vi "Access Privilege_DeleteUser.vi"(8 "error in":errorcluster, 9 "File Path":path, 10 "Username":string, 11 "User ID Refnum":refnum<vi>) -> (0 "error out":errorcluster, 3 "Message Output":string)   [LabVIEW 2023, in "GUI.lvlib"]
doc: "This VI shall delete the selected user on confirmation"
uses:
  GUI.lvlib
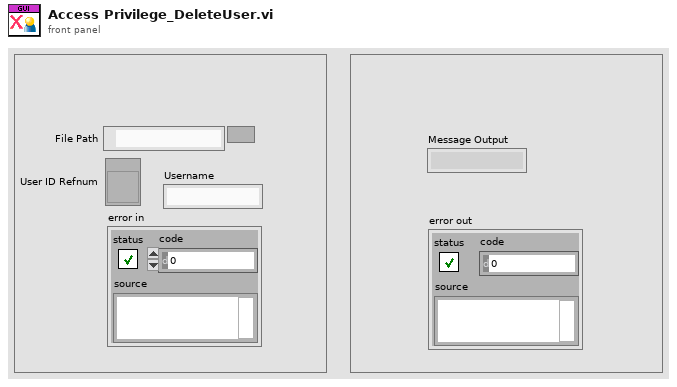
[diagram p1: front panel]
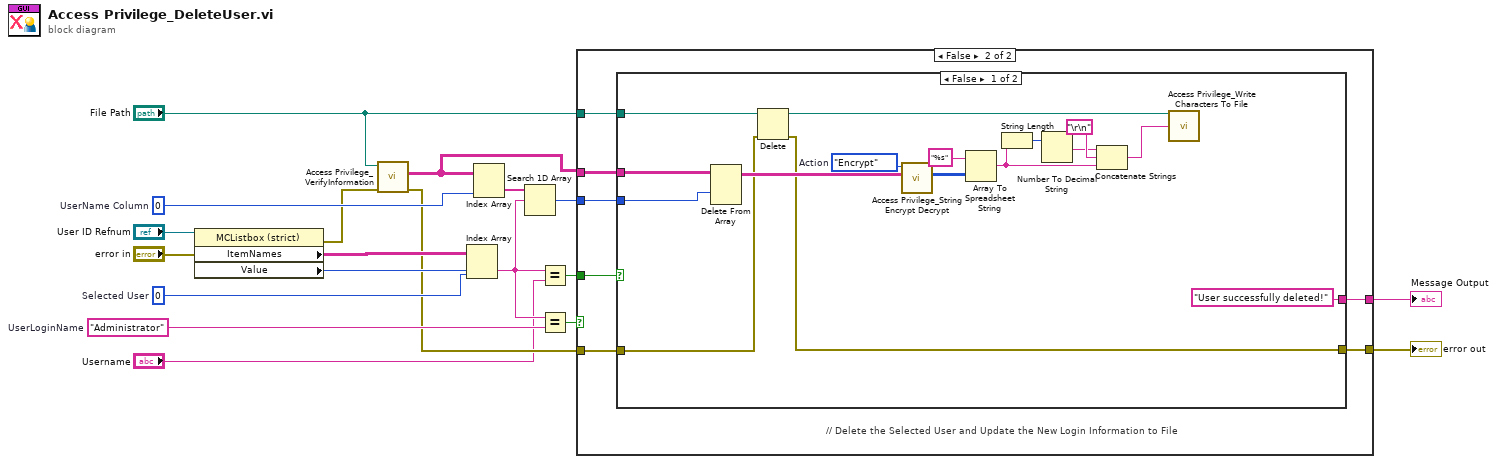
[diagram p0: block diagram]
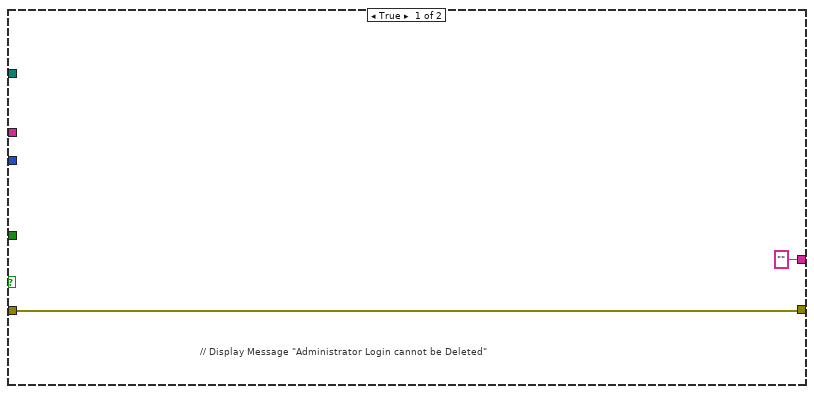
[diagram p2: hidden frame]
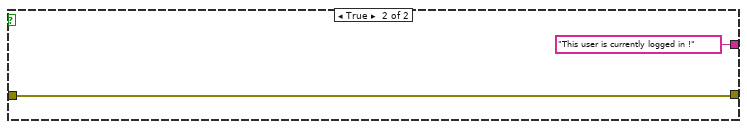
[diagram p3: hidden frame]
diagram:
  w12 = "Administrator"  # UserLoginName
  w14 = 0  # Selected User
  w16 = 0  # UserName Column
  n1 = property class="MCListbox (strict)"(reference="User ID Refnum", error in="error in") -> (error out=w8:errorcluster, "ItemNames"=w17:string[][], "Value"=w18:i32)  [unwired: 1 out]
  n2 = call "Access Privilege_VerifyInformation.vi"("error in (no error)"=w8, "Login Path"="File Path") -> ("error out"=w7:errorcluster, "Login Information"=w6:string[][])  [unwired: 7 in, 1 out]
  n3 = Index Array(array=w17, index (row)=w18, index (col)=w14) -> (element=w3:string)
  n4 = Index Array(array=w6, index (col)=w16) -> (element=w15:string[])  [unwired: 1 in]
  n5 = Search 1D Array(1D array=w15, element=w3) -> (index of element=w11:i32)  [unwired: 1 out]
  n6 = Equal?(x=w3, y="Username") -> (x = y?=w2:bool)
  n7 = Equal?(x=w3, y=w12) -> (x = y?=w4:bool)
  n8 = case shown="False" w4 {
    tunnel: w6 -> [_ w28]
    tunnel: "File Path" -> [_ w26]
    tunnel: w11 -> [_ w27]
    tunnel: w7 -> [w21 w25]
    tunnel: [w21 w24] -> w10
    tunnel: ["" ("List Of Error(s)") w23] -> w5
    tunnel: w2 -> [_ w22]
    frame True {
      # "// Display Message \"Administrator Login cannot be Deleted\""
    }
    frame False {
      # "// Delete the Selected User and Update the New Login Information to File"
      n9 = case shown="False" w22 {
        tunnel: w28 -> [w44 _]
        tunnel: w27 -> [w43 _]
        tunnel: w26 -> [w33 _]
        tunnel: w25 -> [w32 w46]
        tunnel: [w30 w46] -> w24
        tunnel: ["User successfully deleted!" ("List Of Error(s)") "This user is currently logged in !" ("List Of Error(s)")] -> w23
        frame False {
          w40 = enum16{"Encrypt", "Decrypt"}."Encrypt"  # Action
          n10 = Delete From Array(array=w44, index (row)=w43) -> (array with subset deleted=w39:string[][])  [unwired: 2 in, 1 out]
          n11 = Delete(path (use dialog)=w33, error in=w32) -> (deleted path=w31:path, error out=w30:errorcluster)  [unwired: 1 in, 3 out]
          n12 = call "Access Privilege_String Encrypt Decrypt.vi"("2D String Data"=w39, "Action"=w40) -> ("Encrypted Out"=w41:u8[][][])  [unwired: 8 in, 1 out]
          n13 = Array To Spreadsheet String(array=w41, 3:"%s" ("format string")) -> (spreadsheet string=w35:string)  [unwired: 1 out]
          n14 = String Length(string=w35) -> (length=w37:i32)
          n15 = Number To Decimal String(number=w37) -> (decimal integer string=w36:string)  [unwired: 1 out]
          n16 = Concatenate Strings(w36, "\r\n", w35) -> (w34:string)
          n17 = call "Access Privilege_Write Characters To File.vi"("File path (dialog if empty)"=w31, "Character string"=w34) -> ()  [unwired: 13 in, 1 out]
        }
        frame True {
        }
      }
    }
  }
  "error out" <- w10
  "Message Output" <- w5
